vi "Facade 1.vi"(0 "Data In":T4, 2 "Display State In":T2, 3 "Container State":T3) -> (6 "Data Out":T4, 7 "Display State Out":T2, 8 "Action":T1)   [LabVIEW 2011, in "Intellisense Xcontrol.xctl"]
uses:
  Intellisense Xcontrol.xctl
  Data 1.ctl
  <vilib>/_xctls/Container State.ctl
  State 1.ctl
  <vilib>/_xctls/Action.ctl
  <vilib>/event_ctls.llb/eventvkey.ctl
  <vilib>/_xctls/XControlSupport.lvlib
panel:
  in  "String":string
  # "1. Drop the controls that make up the appearance\nof the XControl here.\n\n2. Resize the window to fit the controls\n\n3. If the XControl is of fixed size,  make the \n window not resizable from VI Properties->Window Appearance.\n\n4. If you want the controls to automatically size when the XControl sizes, check  \"Scale all objects on front panel when window resizes\" in File->VI Properties->Window Size page.\n\n5. Show the block diagram and handle events for the controls on this panel."
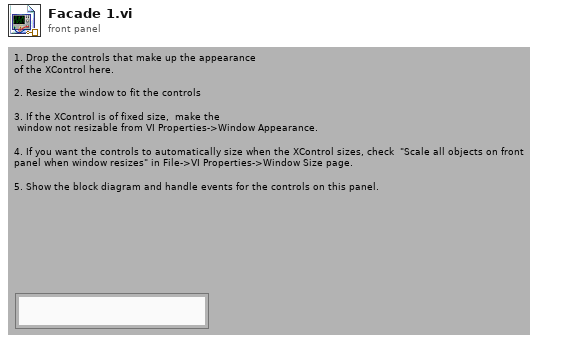
[diagram p1: front panel]
types:
  T1 = typedef "XControlSupport.lvlib/Action.ctl" = cluster{"Data Changed?":bool, "State Changed?":bool, "Action Name":string}
  T2 = typedef "Intellisense Xcontrol.xctl/State 1.ctl" = cluster{"Keyword Array":string[], "Auto-Complete On/Off":bool, "Delimiter":string, "error in (no error)":errorcluster}
  T3 = typedef "XControlSupport.lvlib/Container State.ctl" = cluster{"Indicator?":bool, "Run Mode?":bool, " Refnum":refnum<vi>}
  T4 = typedef "Intellisense Xcontrol.xctl/Data 1.ctl" = string
  T5 = typedef "eventvkey.ctl" = enum16{"ASCII", "Enter", "Return", "Shift", "Ctrl", "Alt", "Cmd", "Opt", "Caps", "NumLock", "Clear", "Break", "Up", "Down", "Left", "Right", "Insert", "Delete", "Home", "End", "PageUp", "PageDown", "Escape", "Help", "Pause", "ScrollLock", "F1", "F2", "F3", "F4", "F5", "F6", "F7", "F8", "F9", "F10", "F11", "F12", "F13", "F14", "F15", "F16", "F17", "F18", "F19", "F20", "F21", "F22", "F23", "F24", "Play", "VolumeUp", "VolumeDown", "Mute", "Two Byte Char"}
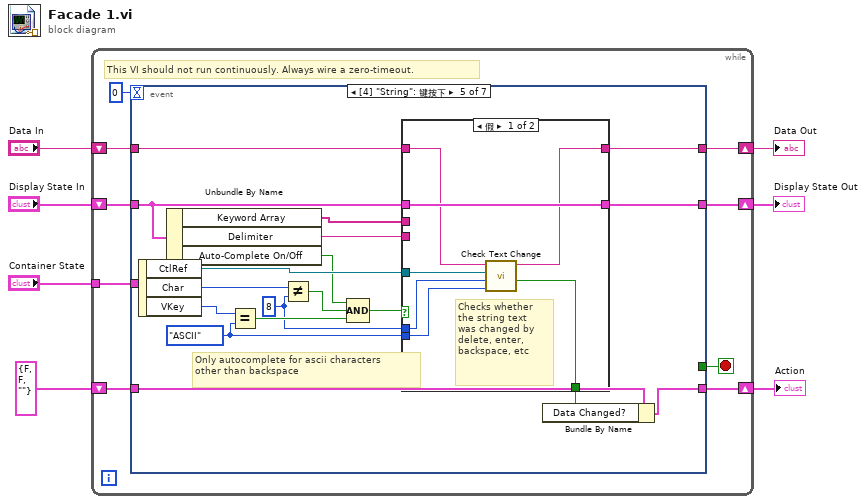
[diagram p0: block diagram]
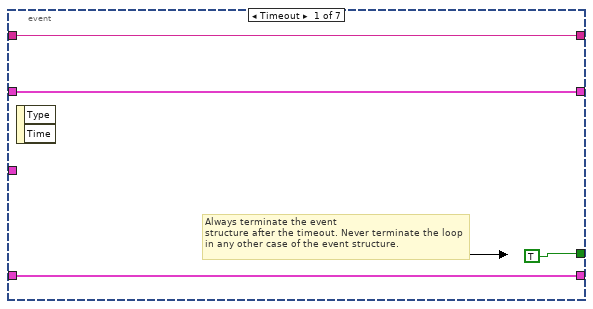
[diagram p2: hidden frame]
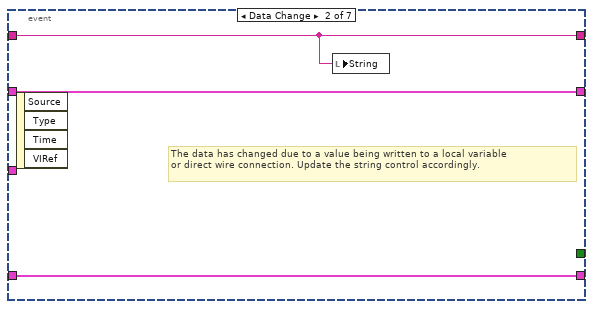
[diagram p3: hidden frame]
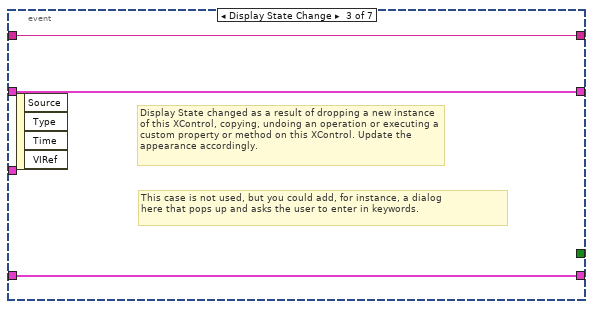
[diagram p4: hidden frame]
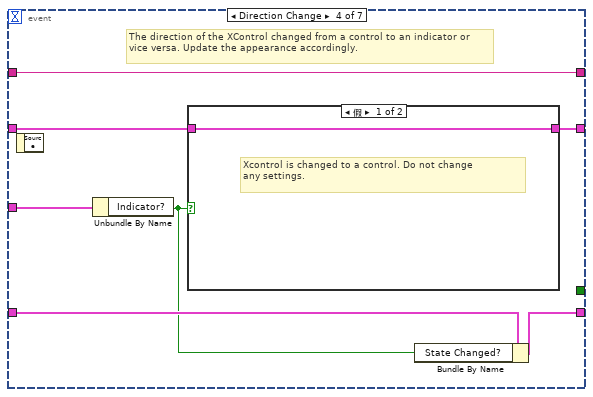
[diagram p5: hidden frame]
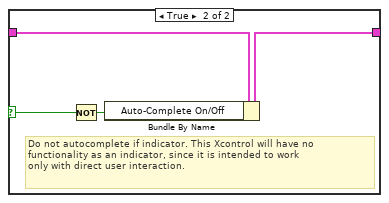
[diagram p6: hidden frame]
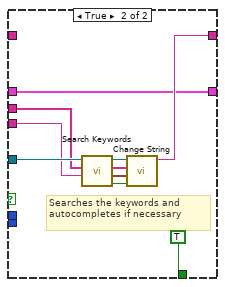
[diagram p7: hidden frame]
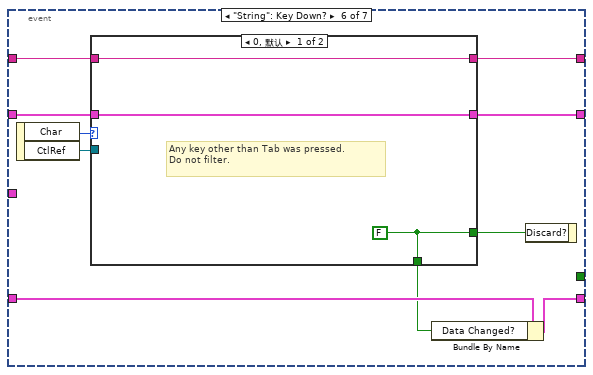
[diagram p8: hidden frame]
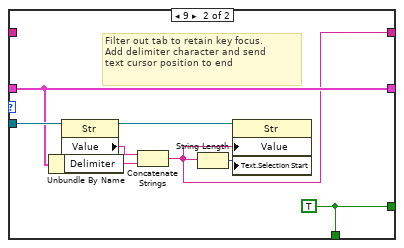
[diagram p9: hidden frame]
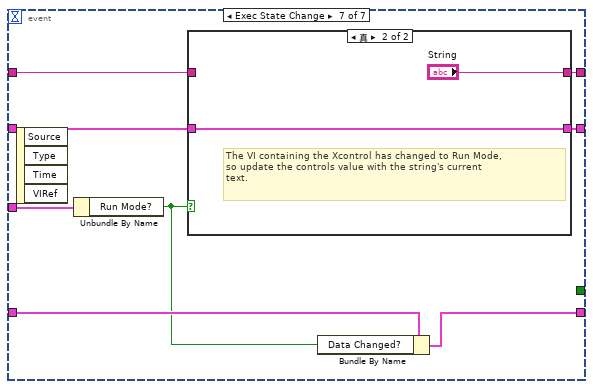
[diagram p10: hidden frame]
diagram:
  n1 = while {
    shift-right: [w15] -> w4
    shift-left: "Display State In" -> [w16]
    tunnel: "Container State" -> [w12]
    shift-right: [w10] -> w7
    shift-left: "Data In" -> [w11]
    shift-right: [w8] -> w2
    shift-left: T1 {"Data Changed?"=FALSE, "State Changed?"=FALSE, "Action Name"=""} ("Action") -> [w9]
    stop <- w14 stop-if-true
    # "This VI should not run continuously. Always wire a zero-timeout."
    n2 = event shown="[4] \"String\": 键按下" {
      selector: _ -> [_ _ _ _ _ _ _]
      dyn-events: _ -> [_ _ _ _ _ _ _]
      timeout: 0 -> [_ _ _ _ _ _ _]
      tunnel: w16 -> [w18 w23 w26 w31 w50 w75 w97]
      tunnel: [w18 w23 w26 w30 w49 w74 w96] -> w15
      tunnel: [TRUE _ _ _ _ _ _] -> w14
      tunnel: w12 -> [_ _ _ w33 _ _ w102]
      tunnel: w11 -> [w17 w21 w25 w32 w48 w77 w98]
      tunnel: [w17 w21 w25 w32 w52 w76 w101] -> w10
      tunnel: [w19 w22 w24 w27 w55 w79 w99] -> w8
      tunnel: w9 -> [w19 w22 w24 w29 w56 w80 w100]
      event Timeout {
        # "Always terminate the event\nstructure after the timeout. Never terminate the loop in any other case of the event structure."
        n3 = event-data() -> ()  [unwired: 1 in, 2 out]
      }
      event Data Change {
        # "The data has changed due to a value being written to a local variable\nor direct wire connection. Update the string control accordingly."
        n4 = event-data() -> ()  [unwired: 1 in, 4 out]
        n5 = local write "String"(w21) -> ()
      }
      event Display State Change {
        # "This case is not used, but you could add, for instance, a dialog\nhere that pops up and asks the user to enter in keywords."
        # "Display State changed as a result of dropping a new instance of this XControl, copying, undoing an operation or executing a custom property or method on this XControl. Update the appearance accordingly."
        n6 = event-data() -> ()  [unwired: 1 in, 4 out]
      }
      event Direction Change {
        # "The direction of the XControl changed from a control to an indicator or vice versa. Update the appearance accordingly."
        n7 = event-data() -> ()  [unwired: 1 in, 1 out]
        n8 = Unbundle By Name(w33) -> ("Indicator?"=w28:bool)
        n9 = case shown="假" w28 {
          selector: w28 -> [_ w35]
          tunnel: w31 -> [w34 w38]
          tunnel: [w34 w36] -> w30
          frame False {
            # "Xcontrol is changed to a control. Do not change\nany settings."
          }
          frame True {
            # "Do not autocomplete if indicator. This Xcontrol will have no\nfunctionality as an indicator, since it is intended to work\nonly with direct user interaction."
            n10 = Not(x=w35) -> (.not. x?=w37:bool)
            n11 = Bundle By Name(cluster=w38, "Auto-Complete On/Off"=w37) -> (w36:T2)
          }
        }
        n12 = Bundle By Name(cluster=w29, "State Changed?"=w28) -> (w27:T1)
      }
      event "String": Key Down {
        w39 = i16 8 ("Char")
        w40 = eventvkey."ASCII" ("VKey")
        # "Only autocomplete for ascii characters\nother than backspace"
        n13 = event-data() -> ("CtlRef"=w54:refnum<vi>, "Char"=w43:i16, "VKey"=w44:T5)  [unwired: 1 in]
        n14 = Unbundle By Name(w50) -> ("Keyword Array"=w53:string[], "Delimiter"=w47:string, "Auto-Complete On/Off"=w46:bool)
        n15 = Equal?(x=w44, y=w40) -> (x = y?=w41:bool)
        n16 = Not Equal?(x=w43, y=w39) -> (x != y?=w42:bool)
        n17 = Compound Arithmetic op=AND(w46, w42, w41) -> (w45:bool)
        n18 = case shown="假" w45 {
          tunnel: w54 -> [w61 w73]
          tunnel: w53 -> [_ w67]
          tunnel: [w60 w71] -> w52
          tunnel: w47 -> [_ w70]
          tunnel: [w57 TRUE ("Data Changed?")] -> w51
          tunnel: w50 -> [w63 w64]
          tunnel: [w63 w64] -> w49
          tunnel: w48 -> [w62 _]
          tunnel: w40 -> [w58 _]
          tunnel: w39 -> [w59 _]
          frame False {
            # "Checks whether\nthe string text\nwas changed by\ndelete, enter,\nbackspace, etc"
            n19 = call "Check Text Change.vi"("VKey"=w58, "Char"=w59, "Str Refnum"=w61, "Data In"=w62) -> ("Text Changed?"=w57:bool, "Data Out"=w60:string)  [unwired: 6 in]
          }
          frame True {
            # "Searches the keywords and\nautocompletes if necessary"
            n20 = call "Search Keywords.vi"("Delimiter"=w70, "Keyword Array"=w67, "Str Refnum"=w73) -> ("Match Found?"=w66:bool, "Match Cluster"=w69:cluster{"Item Index":i32, "Offset":i32}, "Keyword Array Out"=w68:string[], "Str Refnum Out"=w72:refnum<vi>)  [unwired: 5 in]
            n21 = call "Change String.vi"("AutoComplete?"=w66, "Match Cluster"=w69, "Keyword Array"=w68, "String Refnum"=w72) -> ("String Value"=w71:string)  [unwired: 7 in]
          }
        }
        n22 = Bundle By Name(cluster=w56, "Data Changed?"=w51) -> (w55:T1)
      }
      event "String": Key Down? {
        n23 = event-data() -> ("Char"=w83:i16, "CtlRef"=w82:refnum<vi>)  [unwired: 1 in]
        n24 = case shown="0, 默认" w83 {
          tunnel: w82 -> [_ w93]
          tunnel: [w86 w94] -> w81
          tunnel: [w86 w94] -> w78
          tunnel: w77 -> [w85 _]
          tunnel: [w85 w87] -> w76
          tunnel: w75 -> [w84 w89]
          tunnel: [w84 w89] -> w74
          frame 0, Default {
            w86 = FALSE
            # "Any key other than Tab was pressed.\nDo not filter."
          }
          frame 9 {
            w94 = TRUE
            # "Filter out tab to retain key focus.\nAdd delimiter character and send\ntext cursor position to end"
            n25 = Unbundle By Name(w89) -> ("Delimiter"=w88:string)
            n26 = property class="Str"(reference=w93) -> (reference out=w92:refnum<vi>, "Value"=w91:string)  [unwired: 1 in, 1 out]
            n27 = Concatenate Strings(w91, w88) -> (w87:string)
            n28 = String Length(string=w87) -> (length=w90:i32)
            n29 = property class="Str"(reference=w92, "Value"=w87, "Text.Selection Start"=w90) -> ()  [unwired: 1 in, 2 out]
          }
        }
        n30 = Bundle By Name(cluster=w80, "Data Changed?"=w78) -> (w79:T1)
        n31 = event-data("Discard?"=w81) -> ()  [unwired: 1 in, 1 out]
      }
      event Exec State Change {
        n32 = event-data() -> ()  [unwired: 1 in, 4 out]
        n33 = Unbundle By Name(w102) -> ("Run Mode?"=w95:bool)
        n34 = case shown="真" w95 {
          tunnel: [w104 "String"] -> w101
          tunnel: w98 -> [w104 _]
          tunnel: w97 -> [w103 w105]
          tunnel: [w103 w105] -> w96
          frame False {
          }
          frame True {
            # "The VI containing the Xcontrol has changed to Run Mode,\nso update the controls value with the string's current\ntext."
          }
        }
        n35 = Bundle By Name(cluster=w100, "Data Changed?"=w95) -> (w99:T1)
      }
    }
  }
  "Display State Out" <- w4
  "Data Out" <- w7
  "Action" <- w2
